vi "PID Check Step Response.vi"(7 "Norm step factor":dbl, 8 "Length of initial signal":i32, 9 "Initial signal":dbl[](array[numeric]), 10 "Length of tail signal":i32, 11 "tail signal":dbl[](array[numeric])) -> (0 "error code":i32)   [LabVIEW 2017, in "NI_PID_autopid.lvlib"]
uses:
  <vilib>/addons/control/pid/NI_PID_autopid.lvlib
  <vilib>/Analysis/6fits.llb/Curve Fitting Criteria.ctl
  <vilib>/Analysis/NI_AALPro.lvlib
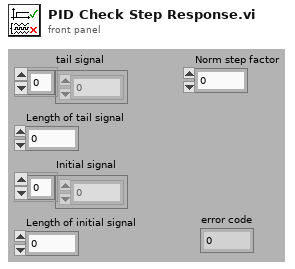
[diagram p1: front panel]
types:
  T1 = typedef "NI_AALPro.lvlib/Curve Fitting Criteria.ctl" = u16
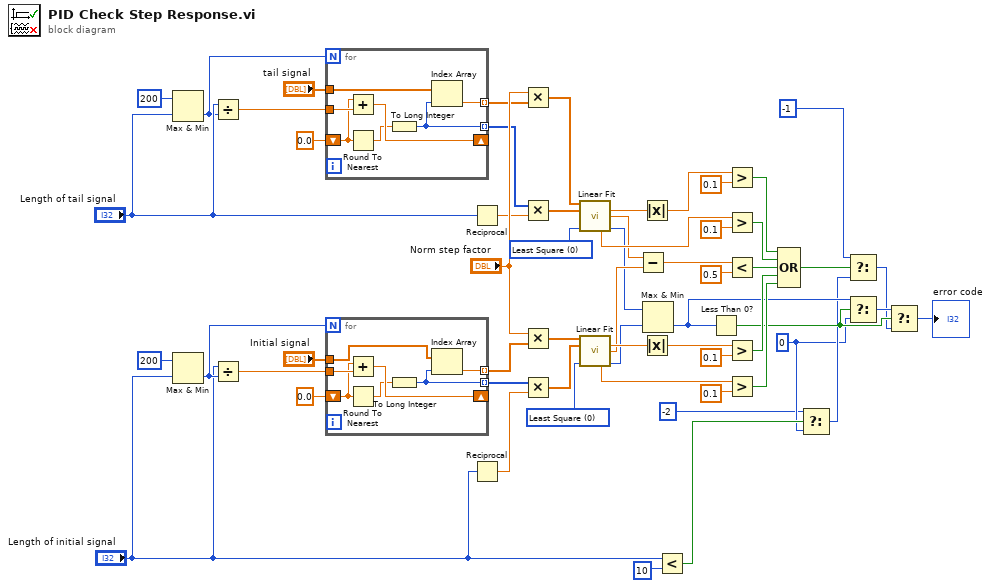
[diagram p0: block diagram]
diagram:
  w2 = 0
  w11 = T1 0 items=["Least Square", "Least Absolute Residual", "Bisquare"] ("method")
  w19 = T1 0 items=["Least Square", "Least Absolute Residual", "Bisquare"] ("method")
  n1 = Max & Min(x=200, y="Length of tail signal") -> (min(x,y)=w55:i32)  [unwired: 1 out]
  n2 = Max & Min(x=200, y="Length of initial signal") -> (min(x,y)=w52:i32)  [unwired: 1 out]
  n3 = Divide(x="Length of tail signal", y=w55) -> (x/y=w13:dbl)
  n4 = Divide(x="Length of initial signal", y=w52) -> (x/y=w5:dbl)
  n5 = for {
    N: w55 -> [_]
    tunnel: "tail signal" -> [w65]
    tunnel: [w64] -> w17 mode=indexing
    shift-right: [w62] -> _
    shift-left: 0.0 ("Signal Length") -> [w61]
    tunnel: w13 -> [w63]
    tunnel: [w59] -> w14 mode=indexing
    n6 = Add(x=w61, y=w63) -> (x+y=w62:dbl)
    n7 = Round To Nearest(number=w61) -> (nearest integer value=w60:dbl)
    n8 = To Long Integer(number=w60) -> (32bit integer=w59:i32)
    n9 = Index Array(array=w65, index=w59) -> (element=w64:dbl)
  }
  n10 = for {
    N: w52 -> [_]
    tunnel: "Initial signal" -> [w72]
    tunnel: [w71] -> w9 mode=indexing
    shift-right: [w69] -> _
    shift-left: 0.0 ("Signal Length") -> [w68]
    tunnel: w5 -> [w70]
    tunnel: [w66] -> w6 mode=indexing
    n11 = Add(x=w68, y=w70) -> (x+y=w69:dbl)
    n12 = Round To Nearest(number=w68) -> (nearest integer value=w67:dbl)
    n13 = To Long Integer(number=w67) -> (32bit integer=w66:i32)
    n14 = Index Array(array=w72, index=w66) -> (element=w71:dbl)
  }
  n15 = Reciprocal(x="Length of tail signal") -> (1/x=w15:dbl)
  n16 = Reciprocal(x="Length of initial signal") -> (1/x=w7:dbl)
  n17 = Multiply(x="Norm step factor", y=w17) -> (x*y=w18:dbl[])
  n18 = Multiply(x=w14, y=w15) -> (x*y=w16:dbl[])
  n19 = Multiply(x="Norm step factor", y=w9) -> (x*y=w10:dbl[])
  n20 = Multiply(x=w6, y=w7) -> (x*y=w8:dbl[])
  n21 = call <vilib>:"Linear Fit.vi"("Y"=w18, "X"=w16, "method"=w19) -> ("slope"=w50:dbl, "intercept"=w40:dbl, "residue"=w45:dbl, "error"=w29:i32)  [unwired: 8 in, 1 out]
  n22 = call <vilib>:"Linear Fit.vi"("Y"=w10, "X"=w8, "method"=w11) -> ("slope"=w49:dbl, "intercept"=w39:dbl, "residue"=w42:dbl, "error"=w28:i32)  [unwired: 8 in, 1 out]
  n23 = Subtract(x=w40, y=w39) -> (x-y=w38:dbl)
  n24 = Absolute Value(x=w50) -> (abs(x)=w48:dbl)
  n25 = Absolute Value(x=w49) -> (abs(x)=w46:dbl)
  n26 = Max & Min(x=w29, y=w28) -> (min(x,y)=w26:i32)  [unwired: 1 out]
  n27 = Less?(x="Length of initial signal", y=10) -> (x < y?=w22:bool)
  n28 = Less Than 0?(x=w26) -> (x < 0?=w25:bool)
  n29 = Greater?(x=w48, y=0.1) -> (0:w36:bool)
  n30 = Greater?(x=w45, y=0.1) -> (0:w35:bool)
  n31 = Less?(x=w38, y=0.5) -> (x < y?=w34:bool)
  n32 = Greater?(x=w46, y=0.1) -> (0:w33:bool)
  n33 = Greater?(x=w42, y=0.1) -> (0:w32:bool)
  n34 = Compound Arithmetic op=OR(w36, w35, w34, w33, w32) -> (w27:bool)
  n35 = Select(t=-2, s=w22, f=w2) -> (s? t:f=w21:i32)
  n36 = Select(t=-1, s=w27, f=w21) -> (s? t:f=w23:i32)
  n37 = Select(t=w26, s=w25, f=w2) -> (s? t:f=w24:i32)
  n38 = Select(t=w24, s=w25, f=w23) -> (s? t:f=→"error code":i32)
